vi "Swerve Begin.vi"(8 "Error In":errorcluster) -> (0 "Error Out":errorcluster)   [LabVIEW 2017]
uses:
  <vilib>/Rock Robotics/SystemInterfaces/DIO/FPGA_DIOChannel.ctl
  Public/Documents/Cross The Road Electronics/Phoenix-LabVIEW/Motor Controller/Controls/CTRE_Phoenix_MotorControl_NeutralMode.ctl
  <vilib>/Rock Robotics/WPI/Counter/WPI_CounterDigitalInputToDigitalSource.vi
  <vilib>/Rock Robotics/WPI/Switch/WPI_SwitchOpenLimit.vi
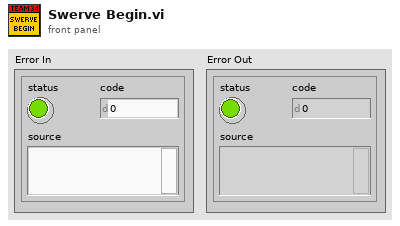
[diagram p1: front panel]
types:
  T1 = typedef "FPGA_DIOChannel.ctl" = enum8{"DIO 0", "DIO 1", "DIO 2", "DIO 3", "DIO 4", "DIO 5", "DIO 6", "DIO 7", "DIO 8", "DIO 9", "DIO MXP 0", "DIO MXP 1", "DIO MXP 2", "DIO MXP 3", "DIO MXP 4", "DIO MXP 5", "DIO MXP 6", "DIO MXP 7", "DIO MXP 8", "DIO MXP 9", "DIO MXP 10", "DIO MXP 11", "DIO MXP 12", "DIO MXP 13", "DIO MXP 14", "DIO MXP 15", "SPI Port CS1", "SPI Port CS2", "SPI Port CS3", "SPI Port MISO", "SPI Port MOSI", "Invalid"}
  T2 = typedef "CTRE_Phoenix_MotorControl_NeutralMode.ctl" = enum8{"EEPROMSetting", "Override to Coast", "Override to Brake"}
  T3 = typedef "WPI_MotorControlDeviceRef.ctl" = cluster{"DeviceStatus":errorcluster, "Type":T4, "PWM":cluster{"PWM Channel":T5, "DeadBand":T6}, "CAN":cluster{"Device Number":u8, "SetOutput VI Ref":variant, "GetOutput VI Ref":variant, "Enable VI Ref":variant, "Disable VI Ref":variant, "Data":variant}, "Invert":bool, "DIO PWM":cluster{"PWM \"Enable\" Channel":T5, "DIOChannel":T1, "PWM Rate":dbl}}
  T4 = typedef "WPI_MotorControlType.ctl" = enum16{"PWM", "CAN", "DIO PWM"}
  T5 = typedef "FPGA_DIOPWMChannel.ctl" = enum8{"PWM 0", "PWM 1", "PWM 2", "PWM 3", "PWM 4", "PWM 5", "PWM 6", "PWM 7", "PWM 8", "PWM 9", "PWM MXP 0", "PWM MXP 1", "PWM MXP 2", "PWM MXP 3", "PWM MXP 4", "PWM MXP 5", "PWM MXP 6", "PWM MXP 7", "PWM MXP 8", "PWM MXP 9", "Invalid"}
  T6 = typedef "WPI_PWMDeadband.ctl" = cluster{"Name":string, "maxPositivePwm":i32, "minPositivePwm":i32, "centerPwm":i32, "maxNegativePwm":i32, "minNegativePwm":i32, "angularRange":u16}
  T7 = typedef "WPI_SwitchDevRef.ctl" = cluster{"DevStatus":errorcluster, "DIO Channel":T1, "CntIndex":T8, "Normally Closed":bool}
  T8 = typedef "FPGA_CounterCtrSystemIndex.ctl" = enum8{"Ctr 0", "Ctr 1", "Ctr 2", "Ctr 3", "Ctr 4", "Ctr 5", "Ctr 6", "Ctr 7", "Invalid"}
  T9 = typedef "WPI_DigitalInputDevRef.ctl" = cluster{"DevStatus":errorcluster, "DIO Channel":T1}
  T10 = typedef "FPGA_CounterEncoderSourceConvertionLVSourceType.ctl" = cluster{"DevStatus":errorcluster, "AnalogTriggerMode?":bool, "DigitalMode":cluster{"DIO Channel":T11}, "AnalogTriggerMode":cluster{"AnalogTriggerIndex":T12, "OutputType":T13}}
  T11 = typedef "FPGA_DIODigitalSourceChannel.ctl" = enum8{"DIO 0", "DIO 1", "DIO 2", "DIO 3", "DIO 4", "DIO 5", "DIO 6", "DIO 7", "DIO 8", "DIO 9", "DIO MXP 0", "DIO MXP 1", "DIO MXP 2", "DIO MXP 3", "DIO MXP 4", "DIO MXP 5", "DIO MXP 6", "DIO MXP 7", "DIO MXP 8", "DIO MXP 9", "DIO MXP 10", "DIO MXP 11", "DIO MXP 12", "DIO MXP 13", "DIO MXP 14", "DIO MXP 15", "Disabled"}
  T12 = typedef "FPGA_AnalogTriggerIndex.ctl" = enum8{"Trig 0", "Trig 1", "Trig 2", "Trig 3", "Trig 4", "Trig 5", "Trig 6", "Trig 7", "Invalid"}
  T13 = typedef "FPGA_AnalogTriggerOutType.ctl" = enum16{"InWindow", "TriggerState", "Rising", "Falling"}
  T14 = typedef "WPI_EncoderDevRef.ctl" = cluster{"DevStatus":errorcluster, "EncoderIndex":T15, "CounterIndex":T8, "DistancePerCount":dbl, "Decoding Type":T16}
  T15 = typedef "FPGA_EncoderIdx.ctl" = enum8{"Enc 0", "Enc 1", "Enc 2", "Enc 3", "Enc 4", "Enc 5", "Enc 6", "Enc 7", "Invalid"}
  T16 = typedef "WPI_EncoderType.ctl" = enum16{"1x", "2x", "4x"}
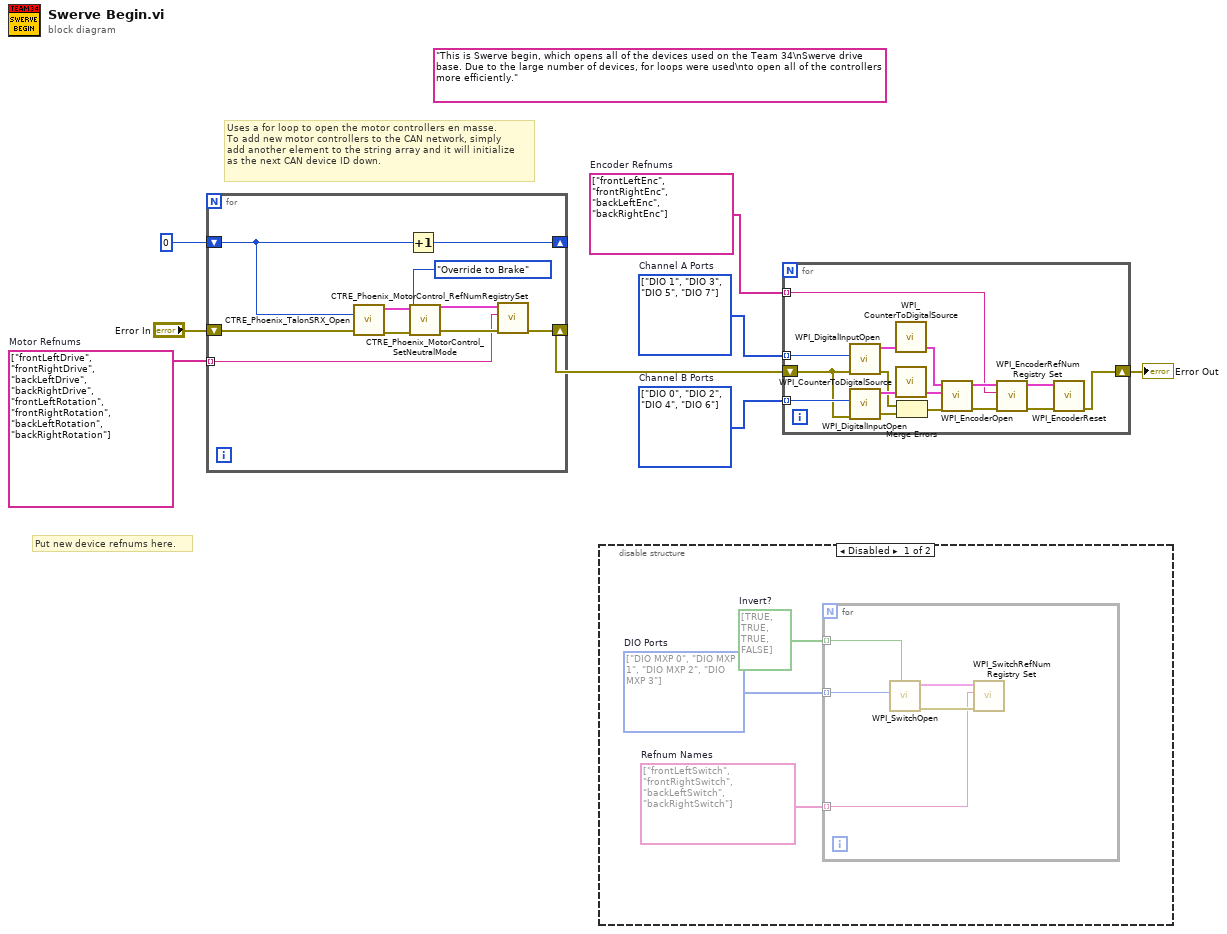
[diagram p0: block diagram]
diagram:
  (unwired) "This is Swerve begin, which opens all of the devices used on the Team 34\nSwerve drive base. Due to the large number of devices, for loops were used\nto open all of the controllers more efficiently."
  w4 = T1[] [enum."DIO 0", enum."DIO 2", enum."DIO 4", enum."DIO 6"] items=["DIO 0", "DIO 1", "DIO 2", "DIO 3", "DIO 4", "DIO 5", "DIO 6", "DIO 7", "DIO 8", "DIO 9", "DIO MXP 0", "DIO MXP 1", "DIO MXP 2", "DIO MXP 3", "DIO MXP 4", "DIO MXP 5", "DIO MXP 6", "DIO MXP 7", "DIO MXP 8", "DIO MXP 9", "DIO MXP 10", "DIO MXP 11", "DIO MXP 12", "DIO MXP 13", "DIO MXP 14", "DIO MXP 15", "SPI Port CS1", "SPI Port CS2", "SPI Port CS3", "SPI Port MISO", "SPI Port MOSI", "Invalid"]  # Channel B Ports
  w5 = T1[] [enum."DIO 1", enum."DIO 3", enum."DIO 5", enum."DIO 7"] items=["DIO 0", "DIO 1", "DIO 2", "DIO 3", "DIO 4", "DIO 5", "DIO 6", "DIO 7", "DIO 8", "DIO 9", "DIO MXP 0", "DIO MXP 1", "DIO MXP 2", "DIO MXP 3", "DIO MXP 4", "DIO MXP 5", "DIO MXP 6", "DIO MXP 7", "DIO MXP 8", "DIO MXP 9", "DIO MXP 10", "DIO MXP 11", "DIO MXP 12", "DIO MXP 13", "DIO MXP 14", "DIO MXP 15", "SPI Port CS1", "SPI Port CS2", "SPI Port CS3", "SPI Port MISO", "SPI Port MOSI", "Invalid"]  # Channel A Ports
  w6 = string[] ["frontLeftEnc", "frontRightEnc", "backLeftEnc", "backRightEnc"]  # Encoder Refnums
  w7 = string[] ["frontLeftDrive", "frontRightDrive", "backLeftDrive", "backRightDrive", "frontLeftRotation", "frontRightRotation", "backLeftRotation", "backRightRotation"]  # Motor Refnums
  # "Put new device refnums here."
  # "Uses a for loop to open the motor controllers en masse.\nTo add new motor controllers to the CAN network, simply\nadd another element to the string array and it will initialize\nas the next CAN device ID down."
  n1 = for {
    shift-right: [w18] -> _
    shift-left: u8 0 -> [w16]
    tunnel: w7 -> [w10] mode=indexing
    shift-right: [w9] -> w3
    shift-left: "Error In" -> [w17]
    n2 = call "CTRE_Phoenix_TalonSRX_Open.vi"("error in"=w17, "Device Number"=w16) -> ("error out"=w13:errorcluster, "CAN Talon SRX Ref"=w14:T3)  [unwired: 8 in]
    n3 = Increment(x=w16) -> (x+1=w18:u8)
    n4 = call "CTRE_Phoenix_MotorControl_SetNeutralMode.vi"("error in (no error)"=w13, "Motor Control Neutral Mode"=CTRE_Phoenix_MotorControl_NeutralMode."Override to Brake", "PhoenixMotorControlDevRef"=w14) -> ("error out"=w11:errorcluster, "PhoenixMotorControlDevRef"=w12:T3)  [unwired: 7 in]
    n5 = call "CTRE_Phoenix_MotorControl_RefNumRegistrySet.vi"("error in (no error)"=w11, "refnum name"=w10, "PhoenixMotorControlDevRef"=w12) -> ("error out"=w9:errorcluster)  [unwired: 7 in, 1 out]
  }
  n6 = disable-structure shown="Disabled" {
    frame Disabled {
      w19 = bool[] [TRUE, TRUE, TRUE, FALSE]  # Invert?
      w20 = T1[] [enum."DIO MXP 0", enum."DIO MXP 1", enum."DIO MXP 2", enum."DIO MXP 3"] items=["DIO 0", "DIO 1", "DIO 2", "DIO 3", "DIO 4", "DIO 5", "DIO 6", "DIO 7", "DIO 8", "DIO 9", "DIO MXP 0", "DIO MXP 1", "DIO MXP 2", "DIO MXP 3", "DIO MXP 4", "DIO MXP 5", "DIO MXP 6", "DIO MXP 7", "DIO MXP 8", "DIO MXP 9", "DIO MXP 10", "DIO MXP 11", "DIO MXP 12", "DIO MXP 13", "DIO MXP 14", "DIO MXP 15", "SPI Port CS1", "SPI Port CS2", "SPI Port CS3", "SPI Port MISO", "SPI Port MOSI", "Invalid"]  # DIO Ports
      w21 = string[] ["frontLeftSwitch", "frontRightSwitch", "backLeftSwitch", "backRightSwitch"]  # Refnum Names
      n7 = for {
        tunnel: w21 -> [w24] mode=indexing
        tunnel: w20 -> [w23] mode=indexing
        tunnel: w19 -> [w22] mode=indexing
        n8 = call-poly <vilib>:"WPI_SwitchOpen.vi"("Normally Closed"=w22, "DIO Channel"=w23) -> ("error out"=w26:errorcluster, "SwitchDevRef"=w25:T7)  [unwired: 8 in]
        n9 = call <vilib>:"WPI_SwitchRefNum Registry Set.vi"("error in (no error)"=w26, "refnum name"=w24, "SwitchDevRef"=w25) -> ()  [unwired: 7 in, 2 out]
      }
    }
    frame Enabled {
    }
  }
  n10 = for {
    tunnel: w6 -> [w32] mode=indexing
    tunnel: w5 -> [w34] mode=indexing
    tunnel: w4 -> [w33] mode=indexing
    shift-right: [w27] -> w1
    shift-left: w3 -> [w28]
    n11 = call <vilib>:"WPI_DigitalInputOpen.vi"("error in (no error)"=w28, "DIO Channel"=w34) -> ("error out"=w29:errorcluster, "DigitalInputDevRef"=w37:T9)  [unwired: 8 out]
    n12 = call <vilib>:"WPI_DigitalInputOpen.vi"("error in (no error)"=w28, "DIO Channel"=w33) -> ("error out"=w30:errorcluster, "DigitalInputDevRef"=w36:T9)  [unwired: 8 out]
    n13 = call-poly <vilib>:"WPI_CounterToDigitalSource.vi"("DigitalInputDevRef"=w37) -> ("Digital Source"=w38:T10)  [unwired: 6 out]
    n14 = call-poly <vilib>:"WPI_CounterToDigitalSource.vi"("DigitalInputDevRef"=w36) -> ("Digital Source"=w35:T10)  [unwired: 6 out]
    n15 = Merge Errors(w29, w30) -> (w31:errorcluster)
    n16 = call <vilib>:"WPI_EncoderOpen.vi"("error in (no error)"=w31, "BSource"=w35, "ASource"=w38) -> ("error out"=w39:errorcluster, "EncoderDevRef"=w40:T14)  [unwired: 5 in, 2 out]
    n17 = call <vilib>:"WPI_EncoderRefNum Registry Set.vi"("error in (no error)"=w39, "refnum name"=w32, "EncoderDevRef"=w40) -> ("error out"=w41:errorcluster, "EncoderDevRef"=w42:T14)  [unwired: 7 in]
    n18 = call <vilib>:"WPI_EncoderReset.vi"("error in (no error)"=w41, "EncoderDevRef"=w42) -> ("error out"=w27:errorcluster)  [unwired: 8 in, 1 out]
  }
  "Error Out" <- w1
